vi "Json build cluster and read.vi"() -> ()   [LabVIEW 2018]
uses:
  e0d47ce7-0286-4a2d-ba25-f39111f699d0.vi
  85e5d0a3-41db-4c26-9811-5f67bc220952.vi
  <vilib>/JDP Science/JSONtext/Variant to JSON Text.vi
  <vilib>/JDP Science/JSONtext/JSON text to Variant.vi
  <vilib>/JDP Science/JSONtext/LVClass Serializer/JSONtext LVClass Serializer.lvclass
  <vilib>/JDP Science/JSONtext/JSONtext.lvlib
panel:
  out "Data out":T1
  out "<JSON>":string caption="<JSON>Object"
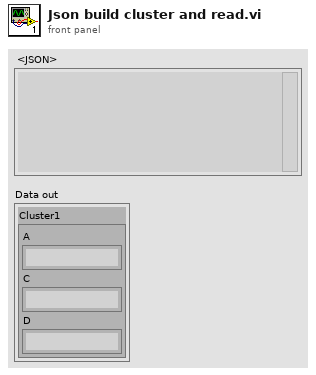
[diagram p1: front panel]
types:
  T1 = cluster{"Cluster1":cluster{"A":string, "C":string, "D":string}}
  T2 = cluster{"Cluster1":cluster{"A":string, "B":string, "C":string}, "Cluster2":cluster{"D":string, "E":string, "F":string}}
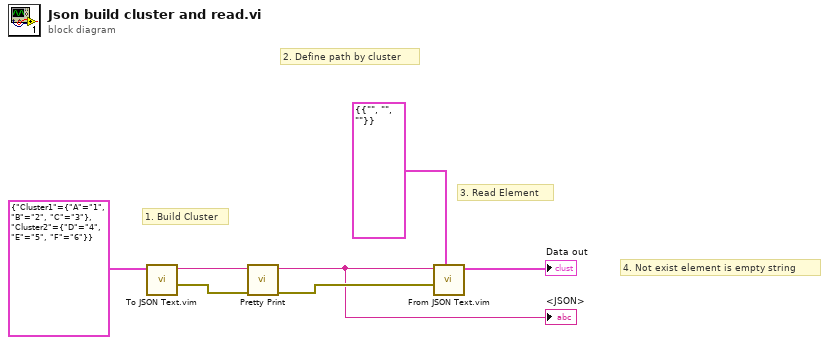
[diagram p0: block diagram]
diagram:
  # "4. Not exist element is empty string"
  # "2. Define path by cluster"
  # "3. Read Element"
  # "1. Build Cluster"
  n1 = call "To JSON Text.vim"("Anything"=T2 {"Cluster1"={"A"="1", "B"="2", "C"="3"}, "Cluster2"={"D"="4", "E"="5", "F"="6"}}) -> ("error out"=w6:errorcluster, "<JSON>"=w7:string)  [unwired: 9 in]
  n2 = call <vilib>:"Pretty Print.vi"("error in (no error)"=w6, "JSON"=w7) -> ("error out"=w5:errorcluster, "<JSON>"=w1:string)  [unwired: 7 in, 1 out]
  "<JSON>" <- w1
  n3 = call "From JSON Text.vim"("Data Type and Default Value"=T1 {"Cluster1"={"A"="", "C"="", "D"=""}}, "error in (no error)"=w5, "JSON"=w1) -> ("Data out"=→"Data out":T1)  [unwired: 7 in, 1 out]
